vi "GetBarHeight.vi"(8 "error in (no error)":errorcluster, 11 "Code39 in":refnum<class "Code39.lvclass">) -> (0 "error out":errorcluster, 2 "Bar Height":u8=25, 3 "Code39 out":refnum<class "Code39.lvclass">)   [LabVIEW 2013, in "BarCodes.lvlib" / "Code39.lvclass"]
uses:
  Code39.lvclass
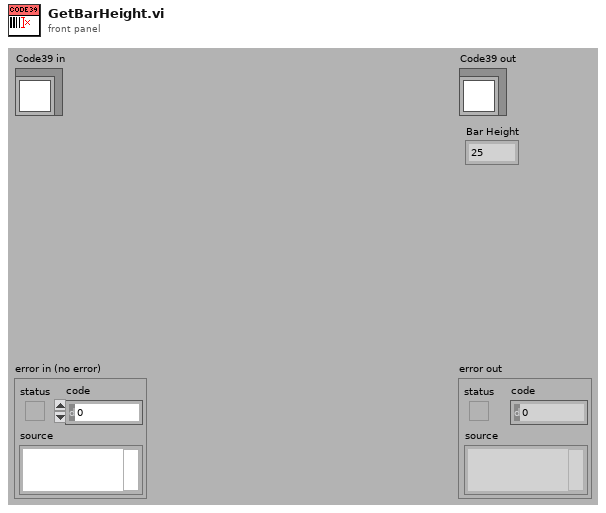
[diagram p1: front panel]
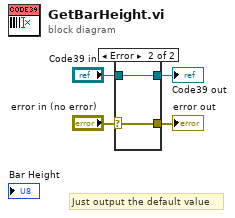
[diagram p0: block diagram]
diagram:
  # "Just output the default value"
  n1 = case shown="Error" "error in (no error)" {
    selector: "error in (no error)" -> [w5 w8]
    tunnel: "Code39 in" -> [w6 w7]
    tunnel: [w6 w7] -> w2
    tunnel: [w5 w8] -> w1
    frame No Error {
    }
    frame Error {
    }
  }
  "error out" <- w1
  "Code39 out" <- w2
